vi "SetConnectionInfo.vi"(7 "LabVIEW Web Service Request":refnum<class "Web Request.lvclass">) -> ()   [LabVIEW 2017]
uses:
  <vilib>/wsapi/Web Request.lvclass
  <vilib>/addons/InsightCM/MessageBus/Base/controls/ConnectionInfo.ctl
  <vilib>/addons/InsightCM/Devices/Shared/Common/ServerComm/ServerComm.lvlib
  <vilib>/addons/Qbus/Qbus.lvclass
panel:
  out "error out":errorcluster
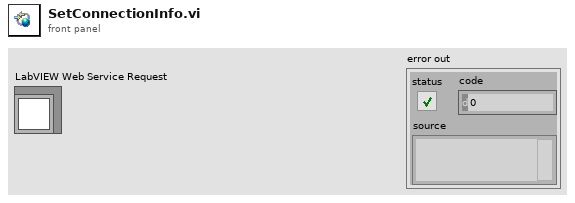
[diagram p1: front panel]
types:
  T1 = typedef "ConnectionInfo.ctl" = cluster{"ClientName":string, "TransceiverHost":string, "TransceiverPort":u16, "Password":string}
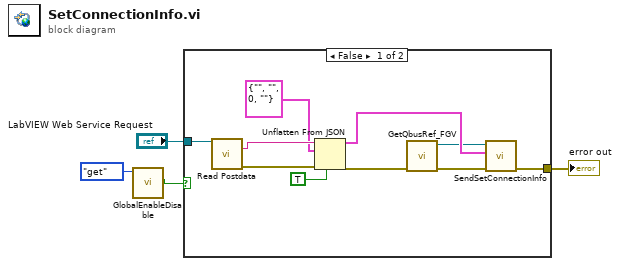
[diagram p0: block diagram]
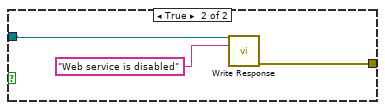
[diagram p2: hidden frame]
diagram:
  n1 = call "GlobalEnableDisable.vi"("action"=enum16{"init", "set", "get"}."get") -> ("DisableDeviceWebService"=w1:bool)  [unwired: 10 in]
  n2 = case shown="False" w1 {
    tunnel: "LabVIEW Web Service Request" -> [w14 w16]
    tunnel: [w9 w15] -> w3
    frame False {
      n3 = call <vilib>:"Read Postdata.vi"("LabVIEW Web Service Request"=w14) -> ("postdata"=w13:string, "error out"=w12:errorcluster)  [unwired: 12 in, 1 out]
      n4 = Unflatten From JSON(JSON string=w13, type and defaults=T1 {"ClientName"="", "TransceiverHost"="", "TransceiverPort"=0, "Password"=""} ("ConnInfo"), default null elements? (F)=TRUE, error in (no error)=w12) -> (value=w10:T1, error out=w6:errorcluster)  [unwired: 3 in]
      n5 = call <vilib>:"GetQbusRef_FGV.vi"("error in (no error)"=w6) -> ("error out"=w7:errorcluster, "Qbus out"=w5:refnum<class "Qbus.lvclass">)  [unwired: 9 in]
      n6 = call <vilib>:"SendSetConnectionInfo.vi"("error in (no error)"=w7, "connection info"=w10, "Qbus in"=w5) -> ("error out"=w9:errorcluster)  [unwired: 7 in, 1 out]
    }
    frame True {
      n7 = call <vilib>:"Write Response.vi"("LabVIEW Web Service Request"=w16, "response string"="Web service is disabled") -> ("error out"=w15:errorcluster)  [unwired: 12 in, 1 out]
    }
  }
  "error out" <- w3
